vi "IsFileNameSafe.vi"(6 "Context":string, 8 "error in (no error)":errorcluster, 11 "candidate":string) -> (0 "error out":errorcluster, 2 "isSafe":bool, 3 "reason":string)   [LabVIEW 2026, in "Lumberjack.lvlib"]
doc: "Pure filename-component predicate. Returns Safe? = FALSE with a Reason when the candidate contains a filesystem-illegal character (< > : \" / \\ | ? *) or a control character; empty is safe (the valid none sentinel for baseName and extension). Dots are legal. Does not raise an error itself; callers (Validate, CreateFileAppender) turn FALSE into config error 5020 with field context. No I/O.\n\nIs a baseName/extension free of filesystem-illegal characters? (empty = safe)"
uses:
  Lumberjack.lvlib
  <vilib>/regexp/Match Regular Expression.xnode
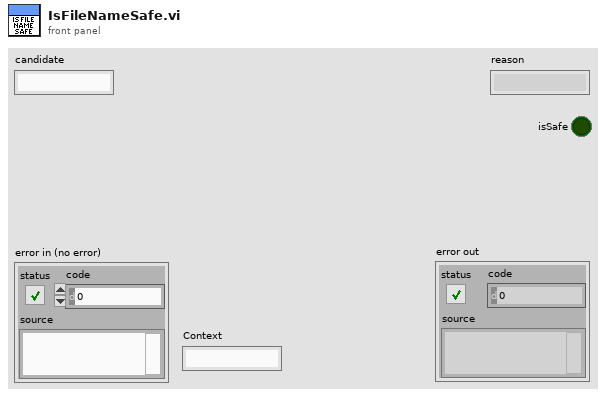
[diagram p1: front panel]
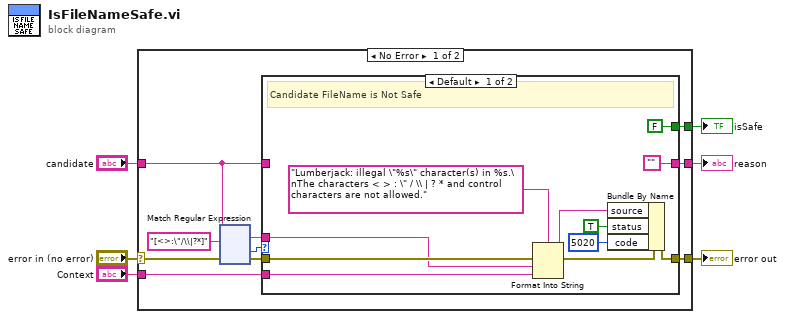
[diagram p0: block diagram]
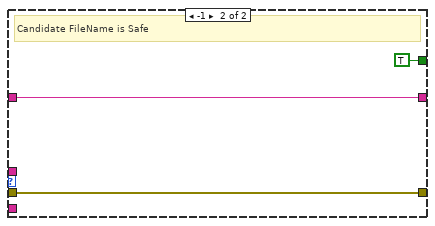
[diagram p2: hidden frame]
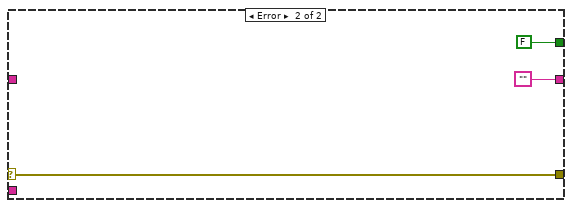
[diagram p3: hidden frame]
diagram:
  n1 = case shown="No Error" "error in (no error)" {
    selector: "error in (no error)" -> [w13 w150]
    tunnel: [w16 w150] -> w5
    tunnel: [w15 FALSE] -> w4
    tunnel: "candidate" -> [w7 _]
    tunnel: [w14 ""] -> w2
    tunnel: "Context" -> [w9 _]
    frame No Error {
      n2 = xnode "Match Regular Expression"("input string"=w7, "regular expression"="[<>:\"/\\|?*]", "error in"=w13) -> ("whole match"=w8:string, "offset past match"=w10:i32, "error out"=w12:errorcluster)  [unwired: 3 in, 2 out]
      n3 = case shown="Default" w10 {
        tunnel: w12 -> [w139 w147]
        tunnel: [w144 w147] -> w16
        tunnel: [FALSE TRUE] -> w15
        tunnel: ["" w145] -> w14
        tunnel: w7 -> [_ w145]
        tunnel: w9 -> [w135 _]
        tunnel: w8 -> [w134 _]
        frame Default {
          # "Candidate FileName is Not Safe"
          n4 = Format Into String(format string="Lumberjack: illegal \"%s\" character(s) in %s.\nThe characters < > : \" / \\ | ? * and control characters are not allowed." ("source"), error in=w139, w134, w135) -> (resulting string=w136:string, error out=w138:errorcluster)  [unwired: 1 in]
          n5 = Bundle By Name(cluster=w138, "source"=w136, "status"=TRUE, "code"=5020) -> (w144:errorcluster)
        }
        frame -1 {
          # "Candidate FileName is Safe"
        }
      }
    }
    frame Error {
    }
  }
  "error out" <- w5
  "reason" <- w2
  "isSafe" <- w4
